vi "Read measurement.vi"(6 "error in":errorcluster, 7 "byte count":u32, 9 "VISA resource name":refnum<visa-resource-name>) -> (0 "error out":errorcluster, 1 "number":dbl, 2 "Read data":string, 3 "VISA resource name out":refnum<visa-resource-name>)   [LabVIEW 2023, in "Aim TTi 1908P DMM.lvlib"]
uses:
  Aim TTi 1908P DMM.lvlib
  19e38209-455c-425b-9d7c-0b824d84d338.vi
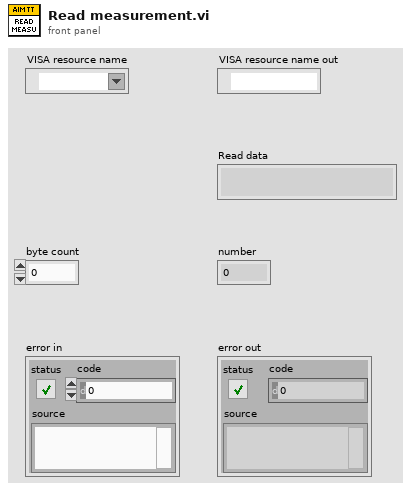
[diagram p1: front panel]
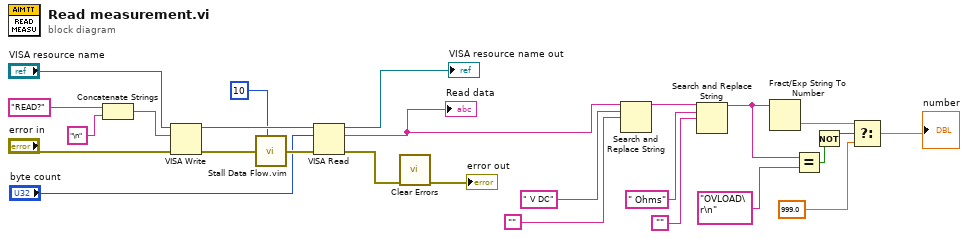
[diagram p0: block diagram]
diagram:
  n1 = Concatenate Strings("READ?" ("Read command"), "\n" ("string")) -> (w19:string)
  n2 = VISA Write(VISA resource name="VISA resource name", write buffer=w19, error in (no error)="error in") -> (VISA resource name out=w26:refnum<visa-resource-name>, error out=w25:errorcluster)  [unwired: 1 out]
  n3 = call "Stall Data Flow.vim"("value in"=w25, "milliseconds to wait"=u32 10) -> ("value out"=w24:errorcluster)  [unwired: 1 out]
  n4 = VISA Read(VISA resource name=w26, byte count="byte count", error in (no error)=w24) -> (VISA resource name out=→"VISA resource name out":refnum<visa-resource-name>, read buffer=w11:string, error out=w16:errorcluster)  [unwired: 1 out]
  "Read data" <- w11
  n5 = call <vilib>:"Clear Errors.vi"("error in (no error)"=w16) -> ("error out"=→"error out":errorcluster)  [unwired: 5 in, 1 out]
  n6 = Search and Replace String(input string=w11, search string=" V DC", replace string="") -> (result string=w10:string)  [unwired: 5 in, 3 out]
  n7 = Search and Replace String(input string=w10, search string=" Ohms", replace string="") -> (result string=w7:string)  [unwired: 5 in, 3 out]
  n8 = Fract/Exp String To Number(string=w7) -> (number=w5:dbl)  [unwired: 3 in, 1 out]
  n9 = Equal?(x=w7, y="OVLOAD\r\n" ("Read data")) -> (x = y?=w4:bool)
  n10 = Not(x=w4) -> (.not. x?=w1:bool)
  n11 = Select(t=w5, s=w1, f=999.0) -> (s? t:f=→"number":dbl)
